vi "open.vi"(0 "object in":refnum<class "serial_work.lvclass">, 1 "input":T1={"IP"="", "PORT"="", "VISA resource name"="", "baud rate (9600)"=115200, "data bits (8)"=8, "parity (0:none)"=enum."None", "timeout (10sec)"=10000} {"data bits (8)" min=5 max=8 step=1}, 5 "error in (no error)":errorcluster) -> (14 "object out":refnum<class "serial_work.lvclass">, 19 "error out":errorcluster)   [LabVIEW 2016, in "serial_work.lvclass"]
uses:
  serial_work.lvclass
  <vilib>/Instr/_visa.llb/VISA Flush IO Buffer Mask.ctl
  serial_work.lvclass/serial_work.ctl
  <vilib>/Instr/_visa.llb/VISA Configure Serial Port (Instr).vi
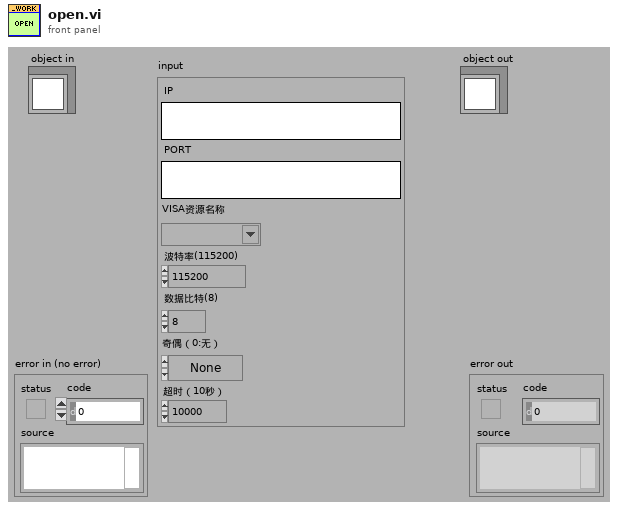
[diagram p1: front panel]
types:
  T1 = cluster{"IP":string, "PORT":string, "VISA resource name":refnum<visa-resource-name>, "baud rate (9600)":u32, "data bits (8)":u16, "parity (0:none)":enum16{"None", "Odd", "Even", "Mark", "Space"}, "timeout (10sec)":u32}
  T2 = typedef "VISA Flush IO Buffer Mask.ctl" = u16
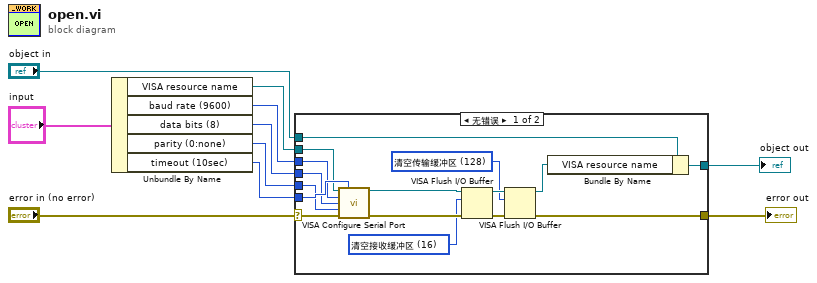
[diagram p0: block diagram]
diagram:
  n1 = Unbundle By Name("input") -> ("VISA resource name"=w1:refnum<visa-resource-name>, "baud rate (9600)"=w5:u32, "data bits (8)"=w4:u16, "parity (0:none)"=w3:enum16{"None", "Odd", "Even", "Mark", "Space"}, "timeout (10sec)"=w2:u32)
  n2 = case shown="无错误" "error in (no error)" {
    selector: "error in (no error)" -> [w13 w28]
    tunnel: [w12 w28] -> w9
    tunnel: [w25 w27] -> w7
    tunnel: "object in" -> [w26 w27]
    tunnel: w2 -> [w17 _]
    tunnel: w5 -> [w16 _]
    tunnel: w4 -> [w15 _]
    tunnel: w3 -> [w14 _]
    tunnel: w1 -> [w11 _]
    frame No Error {
      w19 = T2 128 items=["清空接收缓冲区"=16, "向设备写入传输缓冲区"=32, "清空接收缓冲区（无I/O）"=64, "清空传输缓冲区"=128] ("Mask")
      w22 = T2 16 items=["清空接收缓冲区"=16, "向设备写入传输缓冲区"=32, "清空接收缓冲区（无I/O）"=64, "清空传输缓冲区"=128] ("Mask")
      n3 = call-poly "VISA Configure Serial Port"("VISA resource name"=w11, "timeout (10sec)"=w17, "baud rate (9600)"=w16, "data bits (8)"=w15, "parity (0:none)"=w14, "error in (no error)"=w13) -> ("VISA resource name out"=w23:refnum<visa-resource-name>, "error out"=w24:errorcluster)  [unwired: 8 in]
      n4 = VISA Flush I/O Buffer(VISA resource name=w23, mask (16)=w22, error in (no error)=w24) -> (VISA resource name out=w20:refnum<visa-resource-name>, error out=w21:errorcluster)
      n5 = VISA Flush I/O Buffer(VISA resource name=w20, mask (16)=w19, error in (no error)=w21) -> (VISA resource name out=w18:refnum<visa-resource-name>, error out=w12:errorcluster)
      n6 = Bundle By Name(cluster=w26, "VISA resource name"=w18) -> (w25:refnum<class "serial_work.lvclass">)
    }
    frame Error {
    }
  }
  "error out" <- w9
  "object out" <- w7
